vi "test Get and Set Transceivers.vi"(8 "error in (no error)":errorcluster, 11 "TestCase in":refnum<class "Framework Property Tests.lvclass">) -> (0 "error out":errorcluster, 3 "TestCase out":refnum<class "Framework Property Tests.lvclass">)   [LabVIEW 2017, in "Framework Property Tests.lvclass"]
uses:
  Framework Property Tests.lvclass
  Mock Framework Class/Mock Framework.lvclass
  C:/github/data-sharing-framework/Data Sharing Framework Core/Engine/Classes/Framework/Framework.lvclass
  Engine/Classes/Transceiver/Transceiver.lvclass
  Engine/Classes/Framework/Framework.lvclass/Framework.ctl
  <vilib>/addons/_JKI Toolkits/VI Tester/TestCase.llb/TestCase.lvclass
  Engine/Classes/Framework/Framework.lvclass
  C:/Program Files (x86)/National Instruments/LabVIEW 2017/vi.lib/addons/_JKI Toolkits/VI Tester/TestCase.llb/TestCase.lvclass
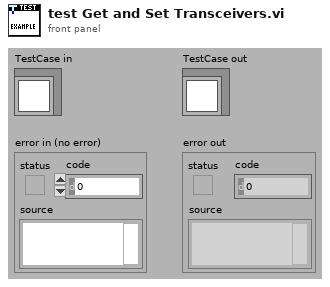
[diagram p1: front panel]
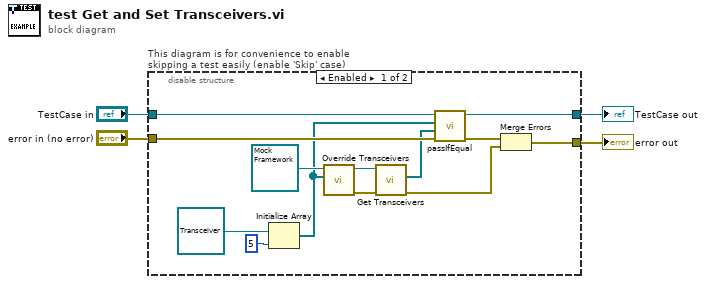
[diagram p0: block diagram]
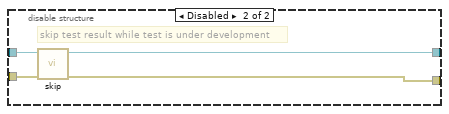
[diagram p2: hidden frame]
diagram:
  n1 = disable-structure "This diagram is for convenience to enable skipping a test easily (enable 'Skip' case)" shown="Enabled" {
    disable-tunnel: "TestCase in" -> [w12 w20]
    disable-tunnel: [w11 w18] -> w1
    disable-tunnel: [w10 w19] -> w3
    disable-tunnel: "error in (no error)" -> [w16 w17]
    frame Enabled {
      n2 = Initialize Array(refnum<class "Transceiver.lvclass"> refnum ("DSF.Engine.lvlib:Transceiver"), 5 ("dimension size")) -> (w8:refnum<class "Transceiver.lvclass">[])
      n3 = call "Override Transceivers.vi"("Transceivers"=w8, "Mock Framework in"=refnum<class "Mock Framework.lvclass"> refnum) -> ("error out"=w9:errorcluster, "Mock Framework out"=w7:refnum<class "Mock Framework.lvclass">)  [unwired: 8 in]
      n4 = call "Get Transceivers.vi"("Framework in"=w7) -> ("Transceivers"=w5:refnum<class "Transceiver.lvclass">[])  [unwired: 9 in, 1 out]
      n5 = call-dynamic "passIfEqual.vi"("error in (no error)"=w16, "y"=w5, "x"=w8, "TestCase in"=w12) -> ("error out"=w13:errorcluster, "TestCase out"=w11:refnum<class "Framework Property Tests.lvclass">)  [unwired: 6 in]
      n6 = Merge Errors(w13, w9) -> (w10:errorcluster)
    }
    frame Disabled {
      # "skip test result while test is under development"
      n7 = call <vilib>:"skip.vi"("error in (no error)"=w17, "TestCase in"=w20) -> ("error out"=w19:errorcluster, "TestCase out"=w18:refnum<class "Framework Property Tests.lvclass">)  [unwired: 8 in]
    }
  }
  "error out" <- w3
  "TestCase out" <- w1
